vi "hamamatsuBufferIndexesAndFrames.vi"   [LabVIEW 2017]
uses:
  globalDevices.vi
  globalUtilities.vi
types:
  T1 = cluster{"height":i32, "width":i32, "datatype":i32}
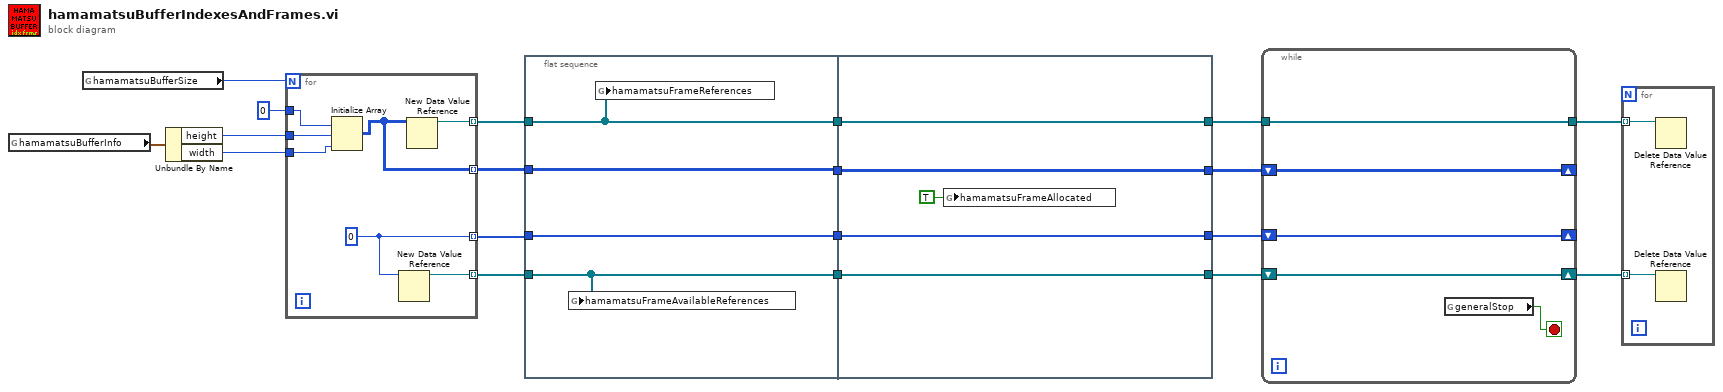
[diagram p0: block diagram]
diagram:
  n1 = global read "globalDevices.vi" "hamamatsuBufferInfo"() -> (w19:T1)
  n2 = global read "globalDevices.vi" "hamamatsuBufferSize"() -> (w8:i32)
  n3 = Unbundle By Name(w19) -> ("height"=w18:i32, "width"=w17:i32)
  n4 = for {
    N: w8 -> [_]
    tunnel: w18 -> [w25]
    tunnel: w17 -> [w24]
    tunnel: u16 0 -> [w26]
    tunnel: [w23] -> w15 mode=indexing
    tunnel: [w22] -> w14 mode=indexing
    tunnel: [w21] -> w3 mode=indexing
    tunnel: [w20] -> w2 mode=indexing
    w21 = 0
    n5 = Initialize Array(w26, w25, w24) -> (w22:u16[][])
    n6 = New Data Value Reference(data value=w21) -> (data value reference=w20:refnum<data-value>)  [unwired: 1 in, 1 out]
    n7 = New Data Value Reference(data value=w22) -> (data value reference=w23:refnum<data-value>)  [unwired: 1 in, 1 out]
  }
  n8 = flat-sequence {
    tunnel: w15 -> [w30]
    tunnel: w14 -> [w29]
    tunnel: [w30] -> w13
    tunnel: [w29] -> w12
    tunnel: [w28] -> w7
    tunnel: w3 -> [w28]
    tunnel: w2 -> [w27]
    tunnel: [w27] -> w5
    tunnel: [w34] -> w10
    tunnel: [w35] -> w11
    tunnel: w13 -> [w35]
    tunnel: w12 -> [w34]
    tunnel: w7 -> [w32]
    tunnel: [w32] -> w6
    tunnel: w5 -> [w31]
    tunnel: [w31] -> w4
    frame #0 {
      n9 = global write "globalDevices.vi" "hamamatsuFrameAvailableReferences"(w27) -> ()
      n10 = global write "globalDevices.vi" "hamamatsuFrameReferences"(w30) -> ()
    }
    frame #1 {
      n11 = global write "globalDevices.vi" "hamamatsuFrameAllocated"(TRUE ("hamamatsuFrameAllocated")) -> ()
    }
  }
  n12 = while {
    tunnel: w11 -> [w39]
    tunnel: [w39] -> w9
    shift-right: [w38] -> _
    shift-left: w10 -> [w38]
    shift-right: [w37] -> _
    shift-left: w6 -> [w37]
    shift-right: [w36] -> w1
    shift-left: w4 -> [w36]
    stop <- w40 stop-if-true
    n13 = global read "globalUtilities.vi" "generalStop"() -> (w40:bool)
  }
  n14 = for {
    tunnel: w9 -> [w42] mode=indexing
    tunnel: w1 -> [w41] mode=indexing
    n15 = Delete Data Value Reference(data value reference=w42) -> ()  [unwired: 1 in, 2 out]
    n16 = Delete Data Value Reference(data value reference=w41) -> ()  [unwired: 1 in, 2 out]
  }
